vi "MecaOdometry_GetKinematics.vi"(11 "in MECA_DRIVE_ODOMETRY":T1={"POSE"={"TRANSLATION"={"X"=0.0, "Y"=0.0}, "ROTATION"={"VALUE"=0.0, "COS"=1.0, "SIN"=0.0}}, "GyroOffset"={"VALUE"=0.0, "COS"=0.0, "SIN"=0.0}, "PreviousAngle"={"VALUE"=0.0, "COS"=0.0, "SIN"=0.0}, "Kinematics"={"FrontLeft"={"X"=0.0, "Y"=0.0}, "FrontRight"={"X"=0.0, "Y"=0.0}, "RearLeft"={"X"=0.0, "Y"=0.0}, "RearRight"={"X"=0.0, "Y"=0.0}, "InverseKinematics"=[[0.0, 1.0, -1.0, 0.0], [0.0, 1.0, 1.0, 0.0], [0.0, 1.0, 1.0, 0.0], [0.0, 1.0, -1.0, 0.0]], "ForwardKinematics"=[[0.0, 1.0, -1.0, 0.0], [0.0, 1.0, 1.0, 0.0], [0.0, 1.0, 1.0, 0.0], [0.0, 1.0, -1.0, 0.0]], "PrevCoR"={"X"=0.0, "Y"=0.0}}, "PreviousWheelPositions"={"FrontLeft"=0.0, "FrontRight"=0.0, "RearLeft"=0.0, "RearRight"=0.0}} {"PreviousWheelPositions"."RearRight" format="%19.3f"; "PreviousWheelPositions"."RearLeft" format="%19.3f"; "PreviousWheelPositions"."FrontRight" format="%19.3f"; "PreviousWheelPositions"."FrontLeft" format="%19.3f"; "Kinematics"."PrevCoR"."Y" format="%14.3f"; "Kinematics"."PrevCoR"."X" format="%14.3f"; "Kinematics"."RearRight"."Y" format="%14.3f"; "Kinematics"."RearRight"."X" format="%14.3f"; "Kinematics"."RearLeft"."Y" format="%14.3f"; "Kinematics"."RearLeft"."X" format="%14.3f"; "Kinematics"."FrontRight"."Y" format="%14.3f"; "Kinematics"."FrontRight"."X" format="%14.3f"; "Kinematics"."FrontLeft"."Y" format="%14.3f"; "Kinematics"."FrontLeft"."X" format="%14.3f"; "PreviousAngle"."SIN" format="%13.4f"; "PreviousAngle"."COS" format="%13.4f"; "PreviousAngle"."VALUE" format="%13.4f"; "GyroOffset"."SIN" format="%13.4f"; "GyroOffset"."COS" format="%13.4f"; "GyroOffset"."VALUE" format="%13.4f"; "POSE"."ROTATION"."SIN" format="%13.4f"; "POSE"."ROTATION"."COS" format="%13.4f"; "POSE"."ROTATION"."VALUE" format="%13.4f"; "POSE"."TRANSLATION"."Y" format="%14.3f"; "POSE"."TRANSLATION"."X" format="%14.3f"}) -> (3 "Mecanum Kinematics":T5={"FrontLeft"={"X"=0.0, "Y"=0.0}, "FrontRight"={"X"=0.0, "Y"=1.0}, "RearLeft"={"X"=0.0, "Y"=0.0}, "RearRight"={"X"=0.0, "Y"=0.0}, "InverseKinematics"=[[0.0, 1.0, -1.0, 0.0], [0.0, 1.0, 1.0, 0.0], [0.0, 1.0, 1.0, 0.0], [0.0, 1.0, -1.0, 0.0]], "ForwardKinematics"=[[0.0, 1.0, -1.0, 0.0], [0.0, 1.0, 1.0, 0.0], [0.0, 1.0, 1.0, 0.0], [0.0, 1.0, -1.0, 0.0]], "PrevCoR"={"X"=0.0, "Y"=0.0}} {"PrevCoR"."Y" format="%14.3f"; "PrevCoR"."X" format="%14.3f"; "RearRight"."Y" format="%14.3f"; "RearRight"."X" format="%14.3f"; "RearLeft"."Y" format="%14.3f"; "RearLeft"."X" format="%14.3f"; "FrontRight"."Y" format="%14.3f"; "FrontRight"."X" format="%14.3f"; "FrontLeft"."Y" format="%14.3f"; "FrontLeft"."X" format="%14.3f"})   [LabVIEW 2019, in "Trajectory_Library.lvlib"]
doc: "Returns the kinematics data cluster for this odometry\n\nParameters:\n - MecaDriveOdometry - Data structure\n\nReturns:\n Mecanum Kinematics - The kinematics data cluster"
uses:
  Trajectory_Library.lvlib
  TypeDef/TRANSLATION2D.ctl
  TypeDef/ROTATION2D.ctl
  TypeDef/POSE2D.ctl
  TypeDef/MECA_DRIVE_ODOMETRY.ctl
  <vilib>/Analysis/Matrix/Datatypes/RealMatrix.ctl
  <vilib>/Analysis/Matrix/NI_Matrix.lvlib
  TypeDef/MECA_DRIVE_KINEMATICS.ctl
  TypeDef/MECA_WHEEL_POSITIONS.ctl
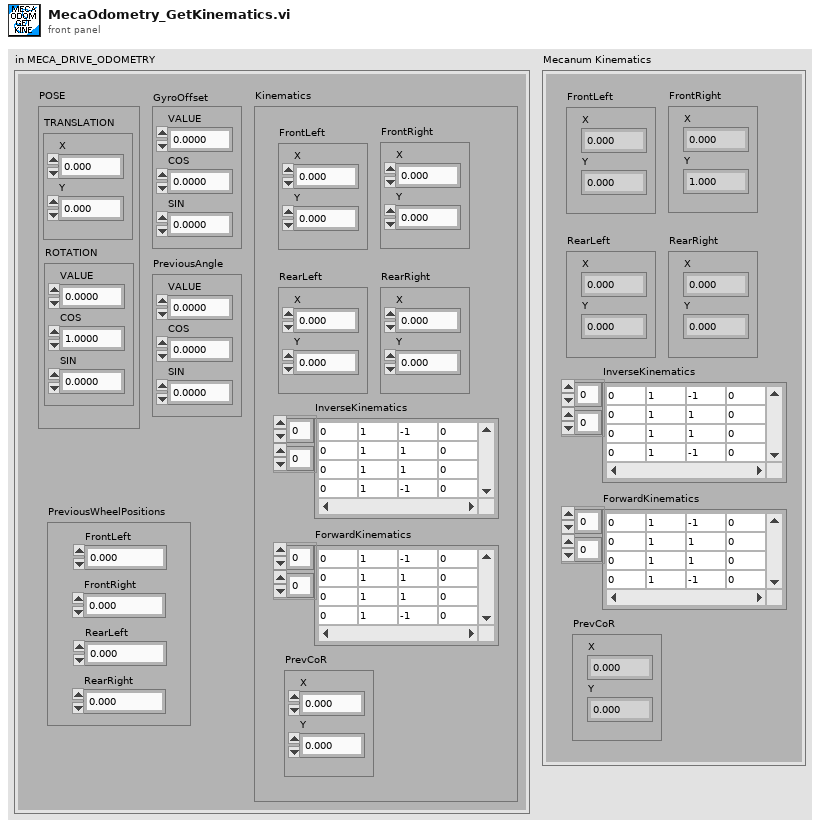
[diagram p1: front panel]
types:
  T1 = typedef "Trajectory_Library.lvlib/MECA_DRIVE_ODOMETRY.ctl" = cluster{"POSE":T2, "GyroOffset":T4, "PreviousAngle":T4, "Kinematics":T5, "PreviousWheelPositions":T7}
  T2 = typedef "Trajectory_Library.lvlib/POSE2D.ctl" = cluster{"TRANSLATION":T3, "ROTATION":T4}
  T3 = typedef "Trajectory_Library.lvlib/TRANSLATION2D.ctl" = cluster{"X":dbl, "Y":dbl}
  T4 = typedef "Trajectory_Library.lvlib/ROTATION2D.ctl" = cluster{"VALUE":dbl, "COS":dbl, "SIN":dbl}
  T5 = typedef "Trajectory_Library.lvlib/MECA_DRIVE_KINEMATICS.ctl" = cluster{"FrontLeft":T3, "FrontRight":T3, "RearLeft":T3, "RearRight":T3, "InverseKinematics":T6, "ForwardKinematics":T6, "PrevCoR":T3}
  T6 = typedef "NI_Matrix.lvlib/RealMatrix.ctl" = dbl[][]
  T7 = typedef "Trajectory_Library.lvlib/MECA_WHEEL_POSITIONS.ctl" = cluster{"FrontLeft":dbl, "FrontRight":dbl, "RearLeft":dbl, "RearRight":dbl}
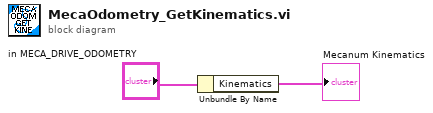
[diagram p0: block diagram]
diagram:
  n1 = Unbundle By Name("in MECA_DRIVE_ODOMETRY") -> ("Kinematics"=→"Mecanum Kinematics":T5)
